vi "subRecursiveSecurityCheck.vi"(8 "error in (no error)":errorcluster, 9 "Blacklist":T1[](array[typedef]), 10 "VI Refnum":refnum<vi>, 11 "CLI":refnum<class "CLI.lvclass">) -> (0 "error out":errorcluster, 1 "Reject?":bool, 2 "dup VI Refnum":refnum<vi>, 3 "CLI out":refnum<class "CLI.lvclass">)   [LabVIEW 2014, in "lvbuildsecurity.lvlib"]
uses:
  lvbuildsecurity.lvlib
  ctlBlacklistClass.ctl
  <vilib>/Wiresmith Technology/LabVIEW CLI/CLI Class/CLI.lvclass
  <vilib>/Utility/traverseref.llb/TRef TravTarget.ctl
  <vilib>/Utility/traverseref.llb/VI Scripting - Traverse.lvlib
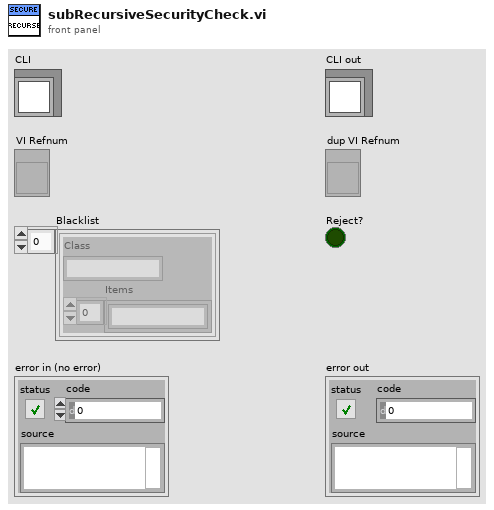
[diagram p1: front panel]
types:
  T1 = typedef "lvbuildsecurity.lvlib/ctlBlacklistClass.ctl" = cluster{"Class":string, "Items":string[]}
  T2 = enum32{"invalid lock state", "Not Locked", "Locked (No Password)", "Password-protected"}
  T3 = typedef "TRef TravTarget.ctl" = enum16{"FP", "BD", "Other"}
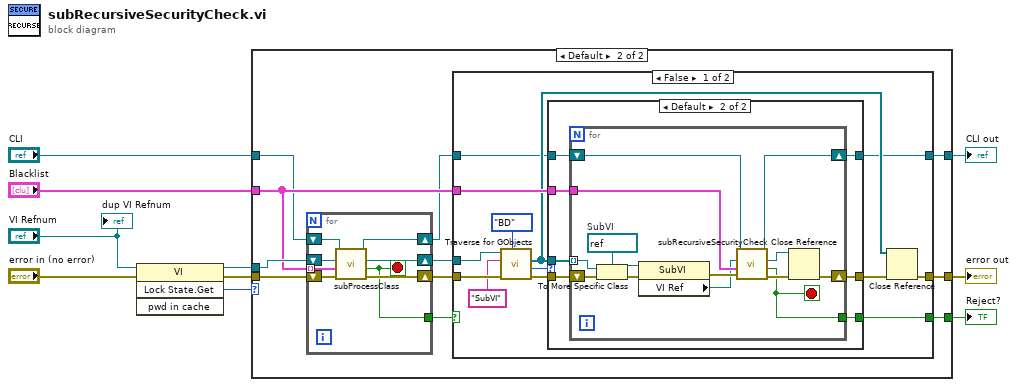
[diagram p0: block diagram]
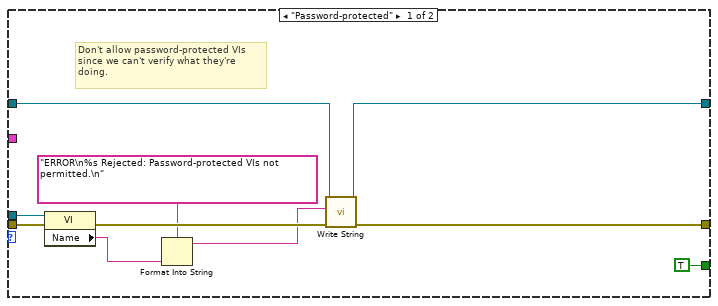
[diagram p2: hidden frame]
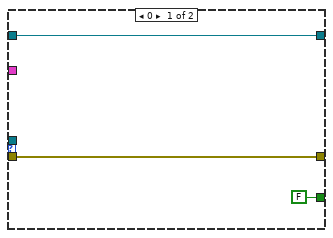
[diagram p3: hidden frame]
diagram:
  n1 = invoke class="VI" method="Lock State.Get"(reference="VI Refnum", error in="error in (no error)") -> (reference out=w9:refnum<vi>, error out=w10:errorcluster, "Get Lock State"=w8:T2)  [unwired: 2 in, 1 out]
  n2 = case shown="Default" w8 {
    tunnel: [w19 w25] -> w6
    tunnel: [TRUE ("Reject?") w26] -> w4
    tunnel: w10 -> [w16 w31]
    tunnel: w9 -> [w15 w30]
    tunnel: "Blacklist" -> [_ w24]
    tunnel: "CLI" -> [w18 w22]
    tunnel: [w17 w23] -> w1
    frame "Password-protected" {
      # "Don't allow password-protected VIs\nsince we can't verify what they're\ndoing."
      n3 = property class="VI"(reference=w15, error in=w16) -> (error out=w14:errorcluster, "Name"=w13:string)  [unwired: 1 out]
      n4 = Format Into String(format string="ERROR\n%s Rejected: Password-protected VIs not permitted.\n", w13) -> (resulting string=w12:string)  [unwired: 2 in, 1 out]
      n5 = call <vilib>:"Write String.vi"("error in (no error)"=w14, "Text to Write"=w12, "CLI in"=w18) -> ("error out"=w19:errorcluster, "CLI out"=w17:refnum<class "CLI.lvclass">)  [unwired: 7 in]
    }
    frame Default {
      n6 = for {
        shift-right: [w78] -> w29
        shift-left: w31 -> [w79]
        tunnel: w24 -> [w75] mode=indexing
        tunnel: [w77] -> w27
        shift-right: [w76] -> w28
        shift-left: w30 -> [w74]
        shift-right: [w72] -> w21
        shift-left: w22 -> [w73]
        stop <- w77 stop-if-true
        n7 = call "subProcessClass.vi"("error in (no error)"=w79, "Blacklist Class"=w75, "VI Refnum"=w74, "CLI"=w73) -> ("error out"=w78:errorcluster, "Reject?"=w77:bool, "dup VI Refnum"=w76:refnum<vi>, "CLI out"=w72:refnum<class "CLI.lvclass">)  [unwired: 4 in]
      }
      n8 = case shown="False" w27 {
        selector: w27 -> [_ w71]
        tunnel: w29 -> [w44 w70]
        tunnel: w28 -> [w43 _]
        tunnel: [w37 w71] -> w26
        tunnel: [w35 w70] -> w25
        tunnel: w24 -> [w36 _]
        tunnel: w21 -> [w33 w69]
        tunnel: [w32 w69] -> w23
        frame False {
          n9 = call <vilib>:"Traverse for GObjects.vi"("Traverse Target"=TRef_TravTarget."BD", "error in (no error)"=w44, "Class Name"="SubVI", "VI Refnum"=w43) -> ("error out"=w39:errorcluster, "# of Refs"=w40:i32, "References"=w34:refnum<vi>[])  [unwired: 4 in, 1 out]
          n10 = case shown="Default" w40 {
            tunnel: w34 -> [_ w52]
            tunnel: w39 -> [w47 w54]
            tunnel: [w47 w53] -> w38
            tunnel: [FALSE ("Reject?") w51] -> w37
            tunnel: w36 -> [_ w50]
            tunnel: w33 -> [w45 w49]
            tunnel: [w45 w48] -> w32
            frame 0 {
            }
            frame Default {
              n11 = for {
                shift-right: [w61] -> w53
                shift-left: w54 -> [w67]
                tunnel: w52 -> [w66] mode=indexing
                tunnel: [w60] -> w51
                tunnel: w50 -> [w59]
                shift-right: [w55] -> w48
                shift-left: w49 -> [w56]
                stop <- w60 stop-if-true
                w65 = refnum<vi> refnum  # SubVI
                n12 = To More Specific Class(target class=w65, reference=w66, error in=w67) -> (specific class reference=w63:refnum<vi>, error out=w64:errorcluster)
                n13 = property class="SubVI"(reference=w63, error in=w64) -> (error out=w62:errorcluster, "VI Ref"=w58:refnum<vi>)  [unwired: 1 out]
                n14 = call "subRecursiveSecurityCheck.vi"("error in (no error)"=w62, "Blacklist"=w59, "VI Refnum"=w58, "CLI"=w56) -> ("error out"=w68:errorcluster, "Reject?"=w60:bool, "dup VI Refnum"=w57:refnum<vi>, "CLI out"=w55:refnum<class "CLI.lvclass">)  [unwired: 4 in]
                n15 = Close Reference(reference=w57, error in (no error)=w68) -> (error out=w61:errorcluster)
              }
            }
          }
          n16 = Close Reference(reference=w34, error in (no error)=w38) -> (error out=w35:errorcluster)
        }
        frame True {
        }
      }
    }
  }
  "error out" <- w6
  "Reject?" <- w4
  "CLI out" <- w1
  "dup VI Refnum" <- "VI Refnum"
